vi "refNewton Raphson Zero Finder user defined derivative.vi"(5 "Variant":variant, 6 "accuracy":dbl=1e-08 format="%.2e", 8 "error in (no error)":errorcluster, 9 "end":dbl=1.0 format="%.2f", 10 "start":dbl format="%.2f", 11 "function refnum":T1) -> (0 "error out":errorcluster, 2 "f(zero)":dbl format="%.2f", 3 "zero":dbl format="%.2f", 4 "f'(zero)":dbl)   [LabVIEW 2017, in "NI_Gmath.lvlib"]
doc: "Determines a zero of a 1D function close to two points with the help of the derivative of this 1D function. The two values form a search limit for the unknown zero of the 1D function."
uses:
  <vilib>/gmath/NI_Gmath.lvlib
  <vilib>/gmath/_ref_NR.llb/functionAndDerivativeRefnum.ctl
panel:
  # "Example:\n\n accuracy: 1E-8 \n h: 1E-8 \n start: 0.0\n end: 1.0\n formula: x^2+sin(x)-1"
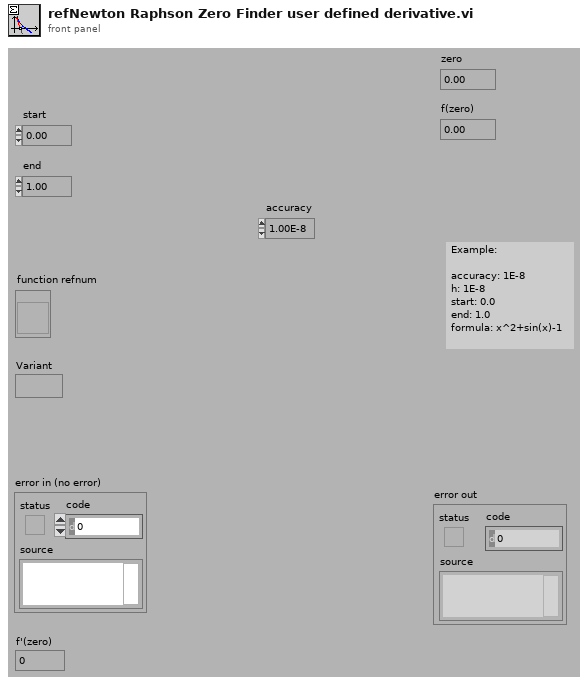
[diagram p1: front panel]
types:
  T1 = typedef "NI_Gmath.lvlib/functionAndDerivativeRefnum.ctl" = refnum<vi>
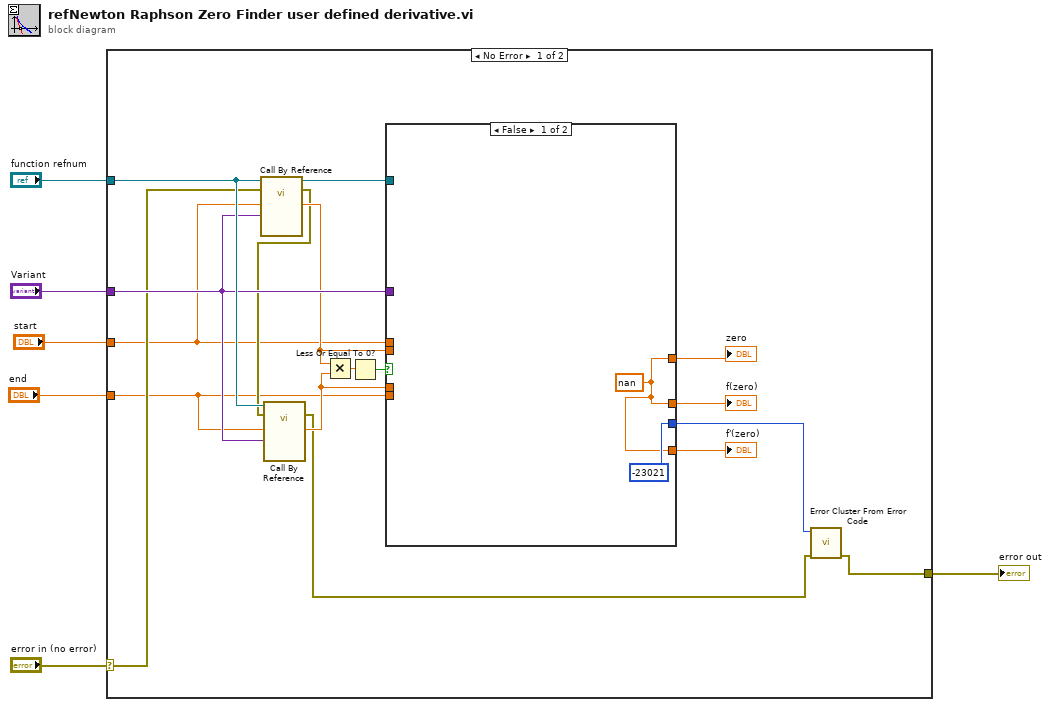
[diagram p0: block diagram]
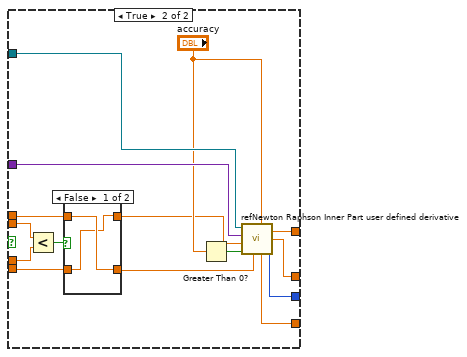
[diagram p2: hidden frame]
diagram:
  n1 = case shown="No Error" "error in (no error)" {
    selector: "error in (no error)" -> [w19 w45]
    tunnel: "function refnum" -> [w21 _]
    tunnel: "Variant" -> [w20 _]
    tunnel: [w10 w45] -> w3
    tunnel: "start" -> [w8 _]
    tunnel: "end" -> [w7 _]
    frame No Error {
      n2 = call-by-ref "?"(reference=w21, error in=w19, "Variant"=w20, "x"=w8) -> (reference out=w15:T1, error out=w12:errorcluster, "f(x)"=w14:dbl)  [unwired: 2 in, 1 out]
      n3 = call-by-ref "?"(reference=w21, error in=w12, "Variant"=w20, "x"=w7) -> (error out=w9:errorcluster, "f(x)"=w13:dbl)  [unwired: 2 in, 2 out]
      n4 = Multiply(x=w14, y=w13) -> (x*y=w16:dbl)
      n5 = Less Or Equal To 0?(x=w16) -> (x <= 0?=w17:bool)
      n6 = case shown="False" w17 {
        tunnel: w8 -> [_ w31]
        tunnel: w7 -> [_ w30]
        tunnel: [w24 w38] -> w23
        tunnel: [w24 w37] -> w22
        tunnel: [-23021 w35] -> w11
        tunnel: w14 -> [_ w29]
        tunnel: w13 -> [_ w28]
        tunnel: w15 -> [_ w40]
        tunnel: w20 -> [_ w39]
        tunnel: [w24 w26] -> w18
        frame False {
          w24 = nan
        }
        frame True {
          n7 = Less?(x=w29, y=w28) -> (x < y?=w34:bool)
          n8 = case shown="False" w34 {
            tunnel: w31 -> [w42 w44]
            tunnel: w30 -> [w41 w43]
            tunnel: [w41 w44] -> w33
            tunnel: [w42 w43] -> w32
            frame False {
            }
            frame True {
            }
          }
          n9 = Greater Than 0?(x="accuracy") -> (x > 0?=w27:bool)
          n10 = call <vilib>:"refNewton Raphson Inner Part user defined derivative.vi"("accuracy"="accuracy", "end/start"=w32, "case"=w27, "start/end"=w33, "Variant"=w39, "function refnum"=w40) -> ("error"=w35:i32, "f'(zero)"=w26:dbl, "zero"=w37:dbl, "f(zero)"=w38:dbl)  [unwired: 1 in]
        }
      }
      "zero" <- w23
      "f(zero)" <- w22
      "f'(zero)" <- w18
      n11 = call <vilib>:"Error Cluster From Error Code.vi"("error in (no error)"=w9, "error code (0)"=w11) -> ("error out"=w10:errorcluster)  [unwired: 7 in]
    }
    frame Error {
    }
  }
  "error out" <- w3
